vi "TSM DAQmx Relays to DAQmx Relay Configuration.vi"(0 "TSM Context":T4, 5 "Relay/Action Connections":T1[](array[typedef]), 11 "error in":errorcluster) -> (4 "DAQmx Relay Configuration Out":T3, 15 "error out":errorcluster)   [LabVIEW 2019]
doc: "Populates the Relay Configuration cluster for the selected relay/action connections. This VI can be used to implement a relay configuration (set of mappings between relay(s) and positions) within a test code module."
uses:
  <vilib>/NI_TestStand_SemiconductorModule/NI_TestStand_Semiconductor_Module.lvlibp/PinMap/General/SemiconductorModuleContext.ctl
  TSM DAQmx Relay Configuration.ctl
  TSM DAQmx Relay to Action Map.ctl
  TSM DAQmx Relay Actions.ctl
  <vilib>/NI_TestStand_SemiconductorModule/NI_TestStand_Semiconductor_Module.lvlibp
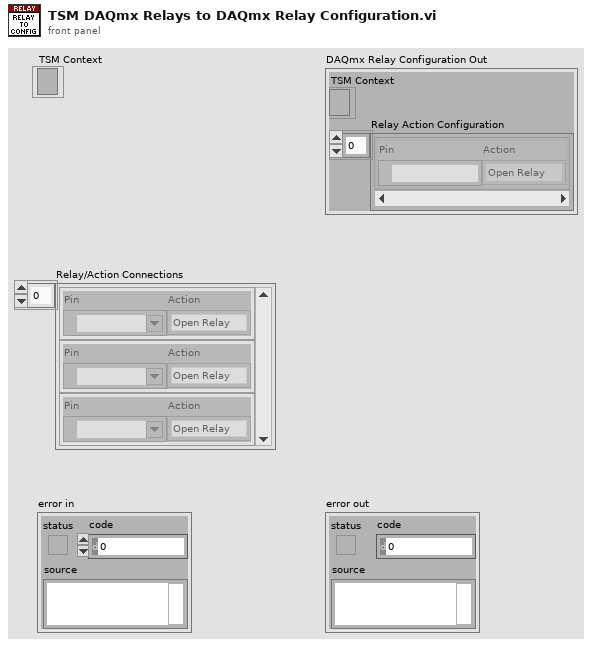
[diagram p1: front panel]
types:
  T1 = typedef "TSM DAQmx Relay to Action Map.ctl" = cluster{"Pin":tag, "Relay Action":T2}
  T2 = typedef "TSM DAQmx Relay Actions.ctl" = enum16{"Open Relay", "Close Relay"}
  T3 = typedef "TSM DAQmx Relay Configuration.ctl" = cluster{"TSM Context":T4, "Relay Action Configuration":T1[]}
  T4 = typedef "NI_TestStand_Semiconductor_Module.lvlibp/SemiconductorModuleContext.ctl" = refnum<k7>
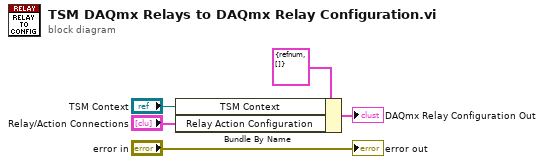
[diagram p0: block diagram]
diagram:
  n1 = Bundle By Name(cluster=T3 {"TSM Context"=refnum, "Relay Action Configuration"=[]} ("TSM SSC Relay Configuration Out 2"), "TSM Context"="TSM Context", "Relay Action Configuration"="Relay/Action Connections") -> (→"DAQmx Relay Configuration Out":T3)
  "error out" <- "error in"
